vi "read_params.vi"(8 "error in (no error)":errorcluster, 11 "LassoLars in":refnum<class "LassoLars.lvclass">) -> (0 "error out":errorcluster, 2 "params":T1={"alpha"=1.0, "fit_intercept"=TRUE, "verbose"={"verbose_type"="bool", "verbose_bool"=FALSE, "verbose_int"=0.0}, "normalize"=TRUE, "precompute"={"precompute_type"="auto", "precompute_bool"=FALSE, "precompute_list"=[]}, "max_iter"=500.0, "copy_X"=TRUE, "fit_path"=TRUE, "positive"=FALSE, "jitter"={"jitter_type"="None", "jitter_float"=0.0}, "random_state"=0.0}, 3 "LassoLars out":refnum<class "LassoLars.lvclass">)   [LabVIEW 2020, in "LassoLars.lvclass"]
uses:
  LassoLars.lvclass
  Controls/lasso_lars_params.ctl
  LassoLars.lvclass/LassoLars.ctl
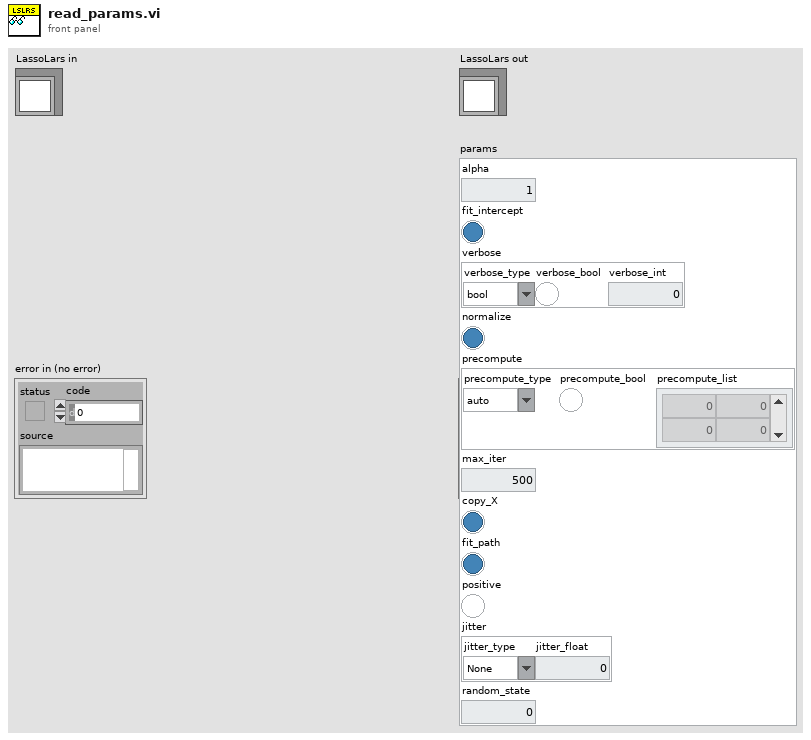
[diagram p1: front panel]
types:
  T1 = typedef "lasso_lars_params.ctl" = cluster{"alpha":dbl, "fit_intercept":bool, "verbose":cluster{"verbose_type":string, "verbose_bool":bool, "verbose_int":dbl}, "normalize":bool, "precompute":cluster{"precompute_type":string, "precompute_bool":bool, "precompute_list":dbl[][]}, "max_iter":dbl, "copy_X":bool, "fit_path":bool, "positive":bool, "jitter":cluster{"jitter_type":string, "jitter_float":dbl}, "random_state":dbl}
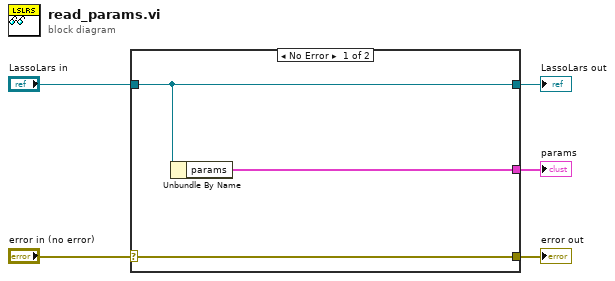
[diagram p0: block diagram]
diagram:
  n1 = case shown="No Error" "error in (no error)" {
    selector: "error in (no error)" -> [w8 w9]
    tunnel: [w8 w9] -> w4
    tunnel: [w7 w10] -> w2
    tunnel: "LassoLars in" -> [w7 w10]
    tunnel: [w6 _] -> w1
    frame No Error {
      n2 = Unbundle By Name(w7) -> ("params"=w6:T1)
    }
    frame Error {
    }
  }
  "error out" <- w4
  "LassoLars out" <- w2
  "params" <- w1
